vi "Continuous.vi"(8 "error in (no error)":errorcluster, 10 "Magnet.lvclass":refnum<class "Magnet.lvclass">, 11 "Continuous.lvclass in":refnum<class "Continuous.lvclass">) -> (0 "error out":errorcluster, 3 "Continuous.lvclass out":refnum<class "Continuous.lvclass">)   [LabVIEW 2009, in "Continuous.lvclass"]
uses:
  Continuous.lvclass
  Instruments/Magnet/Magnet.lvclass
  Scanner/Scanner.lvclass
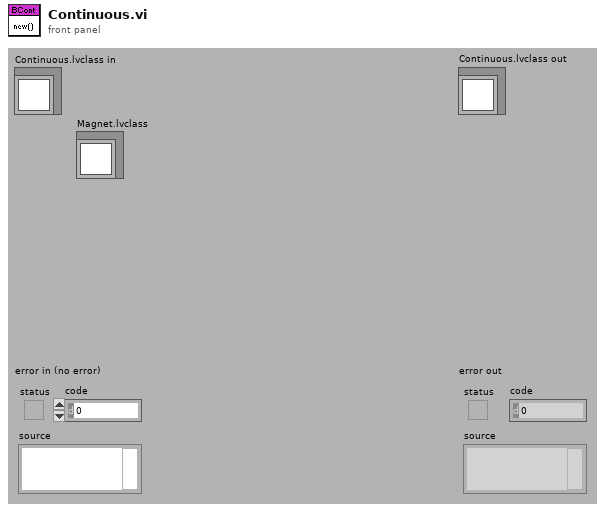
[diagram p1: front panel]
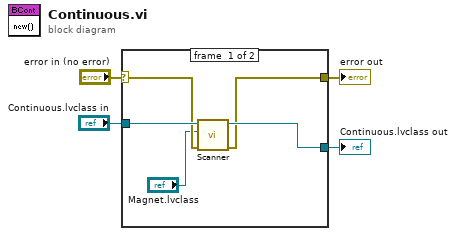
[diagram p0: block diagram]
diagram:
  n1 = case shown="No Error" "error in (no error)" {
    selector: "error in (no error)" -> [w7 w10]
    tunnel: [w6 w10] -> w3
    tunnel: [w8 w11] -> w1
    tunnel: "Continuous.lvclass in" -> [w9 w11]
    frame #0 {
      n2 = call "Scanner.vi"("error in (no error)"=w7, "Scannable"="Magnet.lvclass", "Scanner.lvclass in"=w9) -> ("error out"=w6:errorcluster, "Scanner.lvclass out"=w8:refnum<class "Continuous.lvclass">)  [unwired: 1 in, 6 out]
    }
    frame #1 {
    }
  }
  "error out" <- w3
  "Continuous.lvclass out" <- w1
